vi "Optics_ObtainMessageQueue.vi"(8 "error in (no error)":errorcluster) -> (0 "error out":errorcluster, 3 "Message Queue":refnum<queue>)   [LabVIEW 2021]
doc: "Create a queue with the Message Cluster data type."
uses:
  full-duck/Files/Support/Message Queue/Controls/Message Cluster.ctl
  Controls/Optics_MessageCluster.ctl
  full-duck/Files/Support/Message Queue/Message_queue_library.lvlib
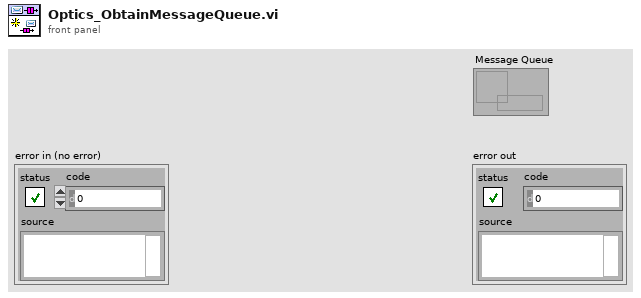
[diagram p1: front panel]
types:
  T1 = typedef "Optics_MessageCluster.ctl" = cluster{"Message":string, "Message Data":variant}
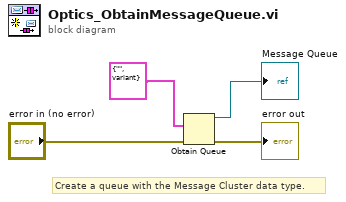
[diagram p0: block diagram]
diagram:
  # "Create a queue with the Message Cluster data type."
  n1 = Obtain Queue(element data type=T1 {"Message"="", "Message Data"=variant} ("Message Cluster"), error in (no error)="error in (no error)") -> (queue out=→"Message Queue":refnum<queue>, error out=→"error out":errorcluster)  [unwired: 3 in, 1 out]
